vi "PH_PSDBWriter.ProcCases.vi"(0 "i ref in":refnum<vi>, 1 "selector":string, 2 "Data":T1, 3 "call cluster":T2={"Object"="", "Selector"="", "CallType"=enum."synchronous", "Async Object"="", "Async Selector"="", "Data Descriptor"="", "Data"=[], "Error #"=0, "Expire"=0}, 5 "error in":errorcluster) -> (14 "i ref out":refnum<vi>, 17 "answer cluster":T2={"Object"="", "Selector"="", "CallType"=enum."synchronous", "Async Object"="", "Async Selector"="", "Data Descriptor"="", "Data"=[], "Error #"=0, "Expire"=0}, 19 "error out":errorcluster)   [LabVIEW 2014, in "PH_PSDBWriter.lvlib"]
doc: "This method is called by a process from within the default case in the event loop. The methods of a class that are linked to events will be called from THIS method. Add your code here."
uses:
  PH_PSDBWriter.lvlib
  CS_Core/CSSystem/CoreDefs/CoreDefs.call_type.ctl
  CS_Core/BaseProcess/BaseProcess.descriptor string definition.ctl
  CS_Core/CSSystem/CoreDefs/CoreDefs.rawDataType.ctl
  PH_PSDBWriter.Thread Commands.ctl
  CS_Core/CSSystem/CoreLib/CoreLib.string 2 byte array.vi
  CS_Core/BaseProcess/BaseProcess.lvlib
  CS_Core/CSSystem/CoreLib/CoreLib.lvlib
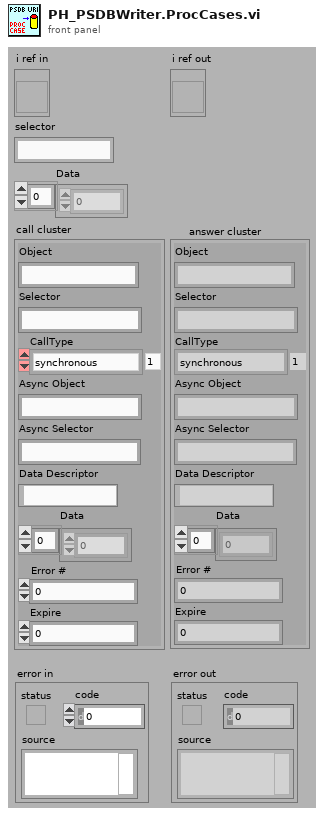
[diagram p1: front panel]
types:
  T1 = typedef "CoreDefs.rawDataType.ctl" = i8[]
  T2 = typedef "CoreDefs.call_type.ctl" = cluster{"Object":string, "Selector":string, "CallType":enum16{"simple", "synchronous", "asynchronous"}, "Async Object":string, "Async Selector":string, "Data Descriptor":T3, "Data":T1, "Error #":i32, "Expire":u32}
  T3 = typedef "BaseProcess.lvlib/BaseProcess.descriptor string definition.ctl" = string
  T4 = typedef "PH_PSDBWriter.lvlib/PH_PSDBWriter.Thread Commands.ctl" = u16
  T5 = typedef "PH_PSDBWriter.lvlib/PH_PSDBWriter.i attribute.ctl" = cluster{"PSDB Status Service ID":i32, "Instance ID":i32, "Shot #":i32, "Subsystem":T6, "Data Status":T7, "Ref PSDB Status":refnum<vi>, "PSDB Error Code":i32, "PSDB Dataset":T8, "PSDB Thread":cluster{"Ref":refnum<vi>, "Q-Ref":refnum<queue>}, "PSDB Credentials":T16}
  T6 = typedef "PH_PSDBWriter.lvlib/PH_PSDBWriter.PHELIX-Subsystems.ctl" = i32
  T7 = typedef "PH_PSDBWriter.lvlib/PH_PSDBWriter.Data Status.ctl" = i16
  T8 = typedef "PH_PSDBWriter.lvlib/PH_PSDBWriter.PSDB Dataset.ctl" = cluster{"Version":i32, "2D data Input":T9[], "Boolean Input":T11[], "Image Input":T12[], "Numeric Input":T14[], "String Input":T15[]}
  T9 = typedef "PH_PSDBWriter.lvlib/PH_PSDBWriter.2D dataset.ctl" = cluster{"name":string, "data":dbl[][], "axis description":T10}
  T10 = typedef "PSDB.lvlib/PSDB_AxisDescription.ctl" = cluster{"x axis label":string, "y axis label":string, "x axis unit":string, "y axis unit":string}
  T11 = typedef "PH_PSDBWriter.lvlib/PH_PSDBWriter.Boolean dataset.ctl" = cluster{"name":string, "data":bool, "unit":string}
  T12 = typedef "PH_PSDBWriter.lvlib/PH_PSDBWriter.Image dataset.ctl" = cluster{"name":string, "data":T13, "unit":string}
  T13 = typedef "IMAQ Image.ctl" = refnum<image>
  T14 = typedef "PH_PSDBWriter.lvlib/PH_PSDBWriter.Numeric dataset.ctl" = cluster{"name":string, "data":dbl, "unit":string}
  T15 = typedef "PH_PSDBWriter.lvlib/PH_PSDBWriter.String dataset.ctl" = cluster{"name":string, "data":string, "unit":string}
  T16 = typedef "PH_Common.lvlib/PH_Connection.PSDB Credentials.ctl" = cluster{"PW":string, "ID":string, "DS":string}
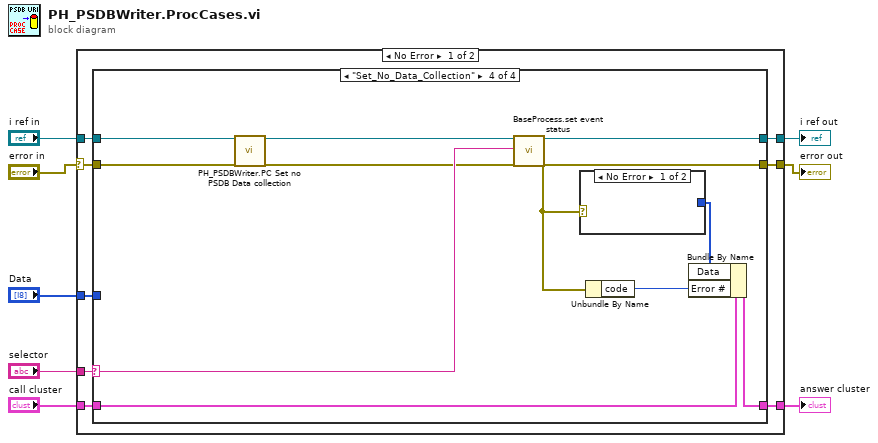
[diagram p0: block diagram]
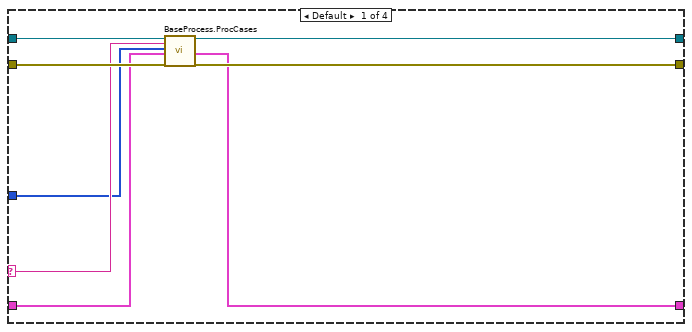
[diagram p2: hidden frame]
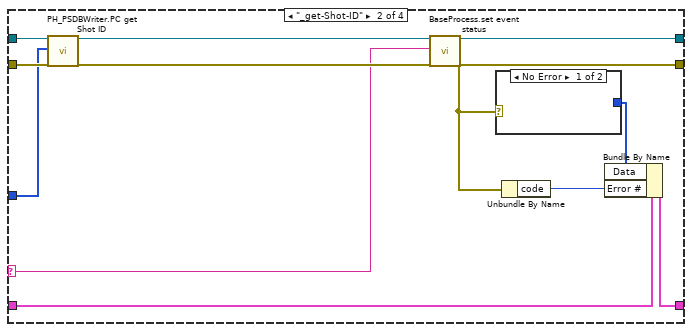
[diagram p3: hidden frame]
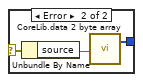
[diagram p4: hidden frame]
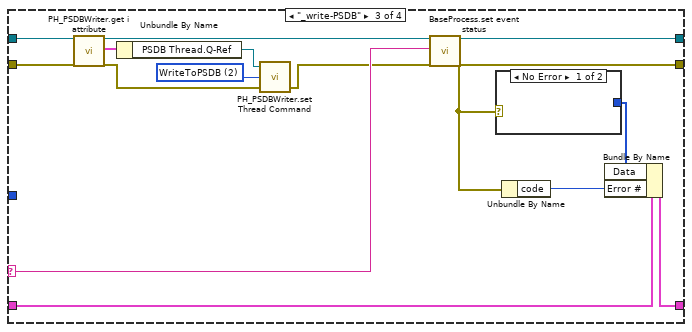
[diagram p5: hidden frame]
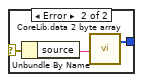
[diagram p6: hidden frame]
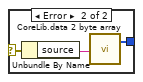
[diagram p7: hidden frame]
diagram:
  n1 = case shown="No Error" "error in" {
    selector: "error in" -> [w9 w73]
    tunnel: "selector" -> [w16 _]
    tunnel: [w15 w72] -> w7
    tunnel: "call cluster" -> [w14 w72]
    tunnel: "i ref in" -> [w13 w74]
    tunnel: [w12 w74] -> w4
    tunnel: [w11 w73] -> w3
    tunnel: "Data" -> [w10 _]
    frame No Error {
      n2 = case shown="\"Set_No_Data_Collection\"" w16 {
        selector: w16 -> [w19 w26 w48 w62]
        tunnel: w10 -> [w17 w25 _ _]
        tunnel: w13 -> [w18 w33 w47 w60]
        tunnel: [w24 w31 w52 w66] -> w12
        tunnel: w14 -> [w20 w27 w49 w63]
        tunnel: [w21 w28 w50 w64] -> w15
        tunnel: w9 -> [w23 w34 w46 w61]
        tunnel: [w22 w29 w51 w65] -> w11
        frame Default {
          n3 = call "BaseProcess.ProcCases.vi"("i ref in"=w18, "selector"=w19, "Data"=w17, "call cluster"=w20, "error in (no error)"=w23) -> ("i ref out"=w24:refnum<vi>, "answer cluster"=w21:T2, "error out"=w22:errorcluster)  [unwired: 12 in]
        }
        frame "_get-Shot-ID" {
          n4 = call "PH_PSDBWriter.PC get Shot ID.vi"("i ref in"=w33, "Data"=w25, "error IO"=w34) -> ("i ref in"=w30:refnum<vi>, "error IO"=w32:errorcluster)  [unwired: 15 in]
          n5 = call "BaseProcess.set event status.vi"("i ref in"=w30, "EventStatus"=w26, "error in (no error)"=w32) -> ("i ref out"=w31:refnum<vi>, "error out"=w29:errorcluster)  [unwired: 14 in, 1 out]
          n6 = case shown="No Error" w29 {
            selector: w29 -> [_ w39]
            tunnel: [_ w37] -> w35
            frame No Error {
            }
            frame Error {
              n7 = Unbundle By Name(w39) -> ("source"=w38:string)
              n8 = call-poly "CoreLib.data 2 byte array.vi"("string"=w38) -> ("byteArray out"=w37:T1)  [unwired: 18 in]
            }
          }
          n9 = Unbundle By Name(w29) -> ("code"=w36:i32)
          n10 = Bundle By Name(cluster=w27, "Data"=w35, "Error #"=w36) -> (w28:T2)
        }
        frame "_write-PSDB" {
          w40 = T4 2 items=["None", "GetInstanceID", "WriteToPSDB"] ("PSDB Thread Command")
          n11 = call "PH_PSDBWriter.get i attribute.vi"("i ref in"=w47, "error in (no error)"=w46) -> ("i ref out"=w45:refnum<vi>, "i attribute"=w42:T5, "error out"=w44:errorcluster)  [unwired: 15 in]
          n12 = Unbundle By Name(w42) -> ("PSDB Thread.Q-Ref"=w41:refnum<queue>)
          n13 = call "PH_PSDBWriter.set Thread Command.vi"("error in (no error)"=w44, "PSDB Thread Command"=w40, "Queue in"=w41) -> ("error out"=w43:errorcluster)  [unwired: 2 in]
          n14 = call "BaseProcess.set event status.vi"("i ref in"=w45, "EventStatus"=w48, "error in (no error)"=w43) -> ("i ref out"=w52:refnum<vi>, "error out"=w51:errorcluster)  [unwired: 14 in, 1 out]
          n15 = case shown="No Error" w51 {
            selector: w51 -> [_ w57]
            tunnel: [_ w55] -> w53
            frame No Error {
            }
            frame Error {
              n16 = Unbundle By Name(w57) -> ("source"=w56:string)
              n17 = call-poly "CoreLib.data 2 byte array.vi"("string"=w56) -> ("byteArray out"=w55:T1)  [unwired: 18 in]
            }
          }
          n18 = Unbundle By Name(w51) -> ("code"=w54:i32)
          n19 = Bundle By Name(cluster=w49, "Data"=w53, "Error #"=w54) -> (w50:T2)
        }
        frame "Set_No_Data_Collection" {
          n20 = call "PH_PSDBWriter.PC Set no PSDB Data collection.vi"("i ref in"=w60, "error IO"=w61) -> ("i ref out"=w59:refnum<vi>, "error out"=w58:errorcluster)  [unwired: 16 in]
          n21 = call "BaseProcess.set event status.vi"("i ref in"=w59, "EventStatus"=w62, "error in (no error)"=w58) -> ("i ref out"=w66:refnum<vi>, "error out"=w65:errorcluster)  [unwired: 14 in, 1 out]
          n22 = case shown="No Error" w65 {
            selector: w65 -> [_ w71]
            tunnel: [_ w69] -> w67
            frame No Error {
            }
            frame Error {
              n23 = Unbundle By Name(w71) -> ("source"=w70:string)
              n24 = call-poly "CoreLib.data 2 byte array.vi"("string"=w70) -> ("byteArray out"=w69:T1)  [unwired: 18 in]
            }
          }
          n25 = Unbundle By Name(w65) -> ("code"=w68:i32)
          n26 = Bundle By Name(cluster=w63, "Data"=w67, "Error #"=w68) -> (w64:T2)
        }
      }
    }
    frame Error {
    }
  }
  "answer cluster" <- w7
  "i ref out" <- w4
  "error out" <- w3
